vi "G#Debugger_AddObject.vi"(0 "Objects dvr":refnum<data-value>, 1 "ObjectInfo":T2, 2 "Ref":refnum<class "G#Object.lvclass">, 5 "error in (no error)":errorcluster) -> (16 "Elements":T1[](array[typedef]), 19 "error out":errorcluster)   [LabVIEW 2017, in "G#Debugger.lvlib"]
uses:
  G#Debugger.lvlib
  G#Object/utils/G#Object_ClassInfoType.ctl
  G#Object/G#Object.lvclass
  G#Object/utils/G#Object_ObjectInfoType.ctl
  G#Object/utils/G#Object_CreateMethod.ctl
  G#Debugger_TreeElement.ctl
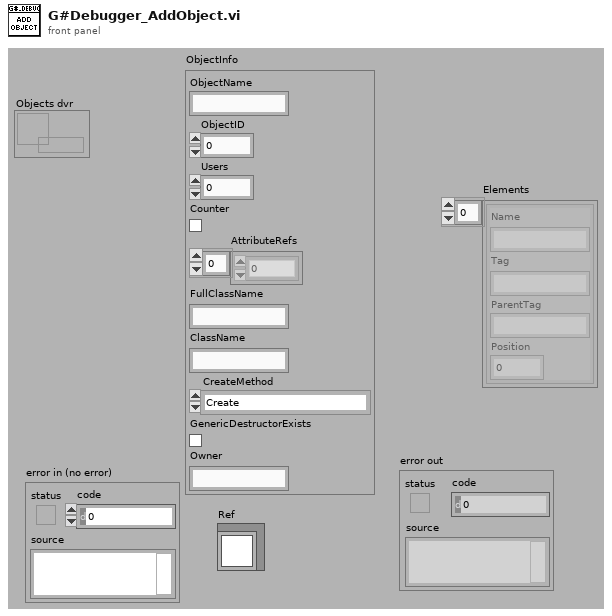
[diagram p1: front panel]
types:
  T1 = typedef "G#Debugger.lvlib/G#Debugger_TreeElement.ctl" = cluster{"Name":string, "Tag":string, "ParentTag":string, "Position":i32}
  T2 = typedef "G#Object.lvclass/G#Object_ObjectInfoType.ctl" = cluster{"ObjectName":string, "ObjectID":u32, "Users":i32, "Counter":bool, "AttributeRefs":u32[], "FullClassName":string, "ClassName":string, "CreateMethod":T3, "GenericDestructorExists":bool, "Owner":string}
  T3 = typedef "G#Object.lvclass/G#Object_CreateMethod.ctl" = enum16{"Create", "Create or look up existing", "Look up existing"}
  T4 = typedef "G#Object.lvclass/G#Object_ClassInfoType.ctl" = cluster{"ClassName":string, "ObjectInfo":T2[], "ObjectRefs":refnum<class "G#Object.lvclass">[], "TypeRef":refnum<class "G#Object.lvclass">}
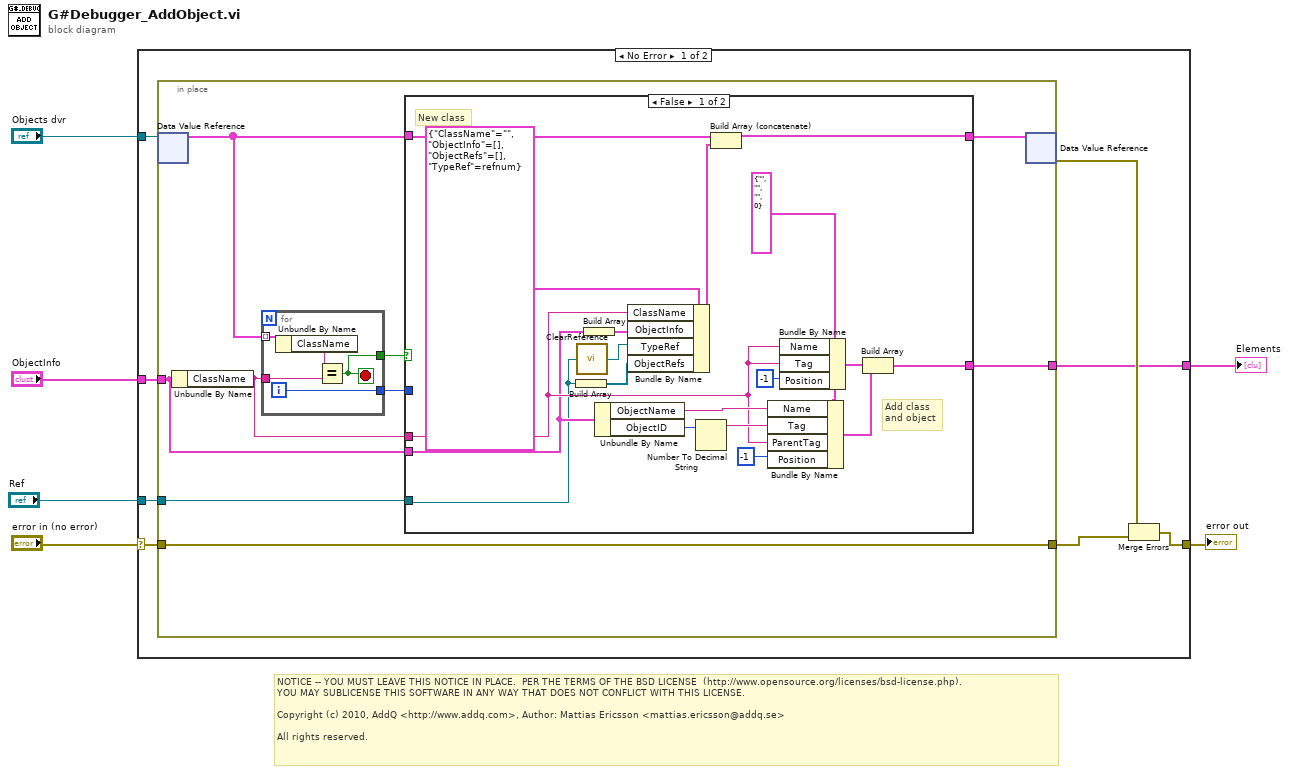
[diagram p0: block diagram]
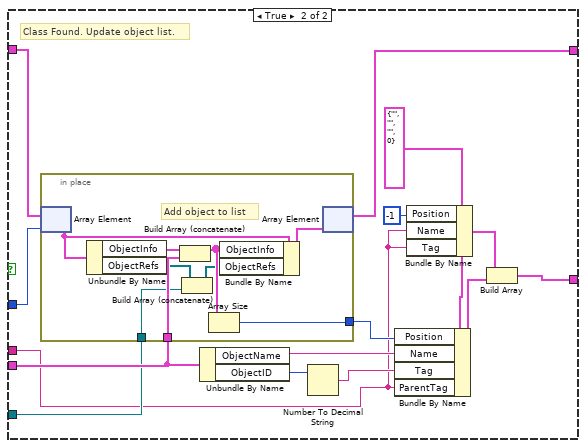
[diagram p2: hidden frame]
diagram:
  # "NOTICE -- YOU MUST LEAVE THIS NOTICE IN PLACE.  PER THE TERMS OF THE BSD LICENSE  (http://www.opensource.org/licenses/bsd-license.php).\nYOU MAY SUBLICENSE THIS SOFTWARE IN ANY WAY THAT DOES NOT CONFLICT WITH THIS LICENSE.\n\nCopyright (c) 2010, AddQ <http://www.addq.com>, Author: Mattias Ericsson <mattias.ericsson@addq.se>\n\nAll rights reserved."
  n1 = case shown="No Error" "error in (no error)" {
    selector: "error in (no error)" -> [w14 w72]
    tunnel: [w12 w72] -> w5
    tunnel: "Objects dvr" -> [w13 _]
    tunnel: "ObjectInfo" -> [w10 _]
    tunnel: [w8 _] -> w2
    tunnel: "Ref" -> [w7 _]
    frame No Error {
      n2 = in-place {
        in-place-border: w14 -> [w17]
        in-place-border: w10 -> [w20]
        in-place-border: [w17] -> w9
        in-place-border: [w16] -> w8
        in-place-border: w7 -> [w15]
        n3 = in-place-dvr #1(w13) -> (w22:T4[])  [unwired: 1 out]
        n4 = Unbundle By Name(w20) -> ("ClassName"=w18:string)
        n5 = for {
          tunnel: w22 -> [w71] mode=indexing
          tunnel: w18 -> [w69]
          tunnel: [w68] -> w21
          tunnel: [w67] -> w23
          i -> [w68]
          stop <- w67 stop-if-true
          n6 = Unbundle By Name(w71) -> ("ClassName"=w70:string)
          n7 = Equal?(x=w70, y=w69) -> (x = y?=w67:bool)
        }
        n8 = case shown="False" w23 {
          tunnel: w22 -> [w42 w57]
          tunnel: w21 -> [_ w55]
          tunnel: w20 -> [w27 w54]
          tunnel: [w39 w56] -> w19
          tunnel: w18 -> [w29 w43]
          tunnel: [w34 w50] -> w16
          tunnel: w15 -> [w25 w47]
          frame False {
            w37 = T1 {"Name"="", "Tag"="", "ParentTag"="", "Position"=0} ("Cluster")
            # "Add class\nand object"
            # "New class"
            n9 = Build Array(w25) -> (w24:refnum<class "G#Object.lvclass">[])
            n10 = call-dynamic "ClearReference.vi"("reference in"=w25) -> ("reference out"=w26:refnum<class "G#Object.lvclass">)
            n11 = Build Array(w27) -> (w38:T2[])
            n12 = Unbundle By Name(w27) -> ("ObjectName"=w33:string, "ObjectID"=w32:u32)
            n13 = Bundle By Name(cluster=T4 {"ClassName"="", "ObjectInfo"=[], "ObjectRefs"=[], "TypeRef"=refnum}, "ClassName"=w29, "ObjectInfo"=w38, "TypeRef"=w26, "ObjectRefs"=w24) -> (w40:T4)
            n14 = Number To Decimal String(number=w32) -> (decimal integer string=w31:string)  [unwired: 1 in]
            n15 = Build Array (concatenate)(w42, w40) -> (w39:T4[])
            n16 = Bundle By Name(cluster=w37, "Name"=w33, "Tag"=w31, "ParentTag"=w29, "Position"=-1) -> (w35:T1)
            n17 = Bundle By Name(cluster=w37, "Name"=w29, "Tag"=w29, "Position"=-1) -> (w36:T1)
            n18 = Build Array(w36, w35) -> (w34:T1[])
          }
          frame True {
            w46 = T1 {"Name"="", "Tag"="", "ParentTag"="", "Position"=0} ("Cluster")
            # "Class Found. Update object list."
            n19 = in-place {
              in-place-border: w54 -> [w66]
              in-place-border: [w62] -> w48
              in-place-border: w47 -> [w58]
              # "Add object to list"
              n20 = in-place-array #2(w57, w55) -> (w65:T4)
              n21 = Unbundle By Name(w65) -> ("ObjectInfo"=w61:T2[], "ObjectRefs"=w60:refnum<class "G#Object.lvclass">[])
              n22 = Build Array (concatenate)(w61, w66) -> (w63:T2[])
              n23 = Build Array (concatenate)(w60, w58) -> (w59:refnum<class "G#Object.lvclass">[])
              n24 = Array Size(array=w63) -> (size(s)=w62:i32)
              n25 = Bundle By Name(cluster=w65, "ObjectInfo"=w63, "ObjectRefs"=w59) -> (w64:T4)
              n26 = in-place-array #2(w64) -> (w56:T4[])  [unwired: 1 out]
            }
            n27 = Unbundle By Name(w54) -> ("ObjectName"=w53:string, "ObjectID"=w52:u32)
            n28 = Number To Decimal String(number=w52) -> (decimal integer string=w51:string)  [unwired: 1 in]
            n29 = Bundle By Name(cluster=w46, "Position"=w48, "Name"=w53, "Tag"=w51, "ParentTag"=w43) -> (w49:T1)
            n30 = Bundle By Name(cluster=w46, "Position"=-1, "Name"=w43, "Tag"=w43) -> (w45:T1)
            n31 = Build Array(w45, w49) -> (w50:T1[])
          }
        }
        n32 = in-place-dvr #1(w19) -> (w11:errorcluster)  [unwired: 1 out]
      }
      n33 = Merge Errors(w11, w9) -> (w12:errorcluster)
    }
    frame Error {
    }
  }
  "error out" <- w5
  "Elements" <- w2
